vi "ROI entry-Initialise image display tools.vi"(8 "error in (no error)":errorcluster) -> (0 "error out":errorcluster)   [LabVIEW 2020]
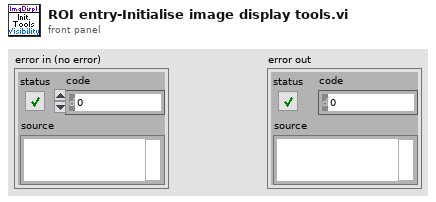
[diagram p1: front panel]
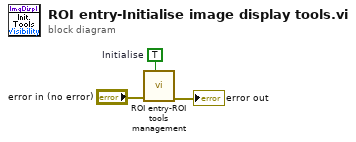
[diagram p0: block diagram]
diagram:
  w3 = TRUE  # Initialise
  n1 = call "ROI entry-ROI tools management.vi"("Initialise"=w3, "error in (no error)"="error in (no error)") -> ("error out"=→"error out":errorcluster)  [unwired: 9 in]
